vi "ResizeCoeffArray.vi"(10 "target size":i32, 11 "Array in":fxp<+/-,18,18>[](array[numeric])) -> (3 "Array out":fxp<+/-,18,18>[](array[numeric]))   [LabVIEW 2013]
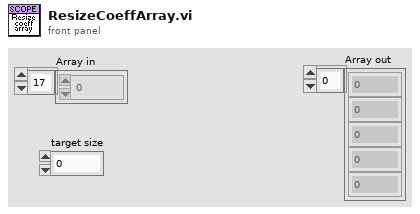
[diagram p1: front panel]
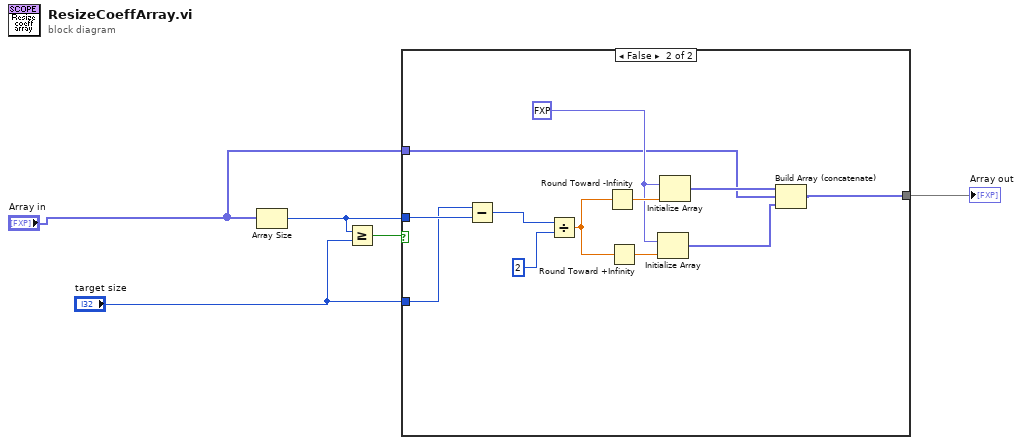
[diagram p0: block diagram]
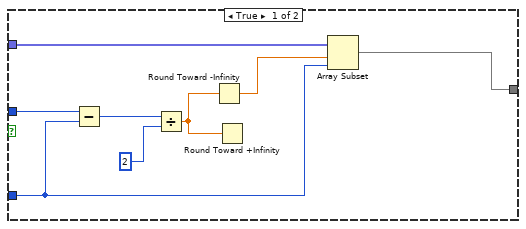
[diagram p2: hidden frame]
diagram:
  n1 = Array Size(array="Array in") -> (size(s)=w5:i32)
  n2 = Greater Or Equal?(x=w5, y="target size") -> (x >= y?=w3:bool)
  n3 = case shown="False" w3 {
    tunnel: [w9 w14] -> w2
    tunnel: "Array in" -> [w8 w16]
    tunnel: w5 -> [w7 w22]
    tunnel: "target size" -> [w6 w21]
    frame True {
      n4 = Subtract(x=w7, y=w6) -> (x-y=w13:i32)
      n5 = Divide(x=w13, y=2) -> (x/y=w11:dbl)
      n6 = Round Toward -Infinity(1:w11) -> (0:w10:dbl)
      n7 = Round Toward +Infinity(x=w11) -> ()  [unwired: 1 out]
      n8 = Array Subset(array=w8, index=w10, length=w6) -> (w9:fxp<+/-,18,18>[])
    }
    frame False {
      w18 = fxp<+/-,18,18> 0.0 ("fixed-point type")
      n9 = Subtract(x=w21, y=w22) -> (x-y=w25:i32)
      n10 = Divide(x=w25, y=2) -> (x/y=w23:dbl)
      n11 = Round Toward -Infinity(1:w23) -> (0:w20:dbl)
      n12 = Round Toward +Infinity(x=w23) -> (ceil(x): smallest int >= x=w19:dbl)
      n13 = Initialize Array(w18, w19) -> (w15:fxp<+/-,18,18>[])
      n14 = Initialize Array(w18, w20) -> (w17:fxp<+/-,18,18>[])
      n15 = Build Array (concatenate)(w17, w16, w15) -> (w14:fxp<+/-,18,18>[])
    }
  }
  "Array out" <- w2
